vi "LabviewV4.vi"() -> ()   [LabVIEW 2010]
uses:
  <vilib>/Instr/_visa.llb/VISA Configure Serial Port (Instr).vi
panel:
  in  "Registar tensão":bool
  in  "Posição de destino da bola (Set Point)":i16
  out "Instruções":string="HOME X Y\r\n" caption="Instruções para traçar gráfico"
  out "Mensagem enviada":string="HOME X Y\r\n"
  out "read string":string caption="Recebido"
  in  "delay before read (ms)":u32=500
  in  "stop":bool
  in  "VISA Resource Name":refnum<visa-resource-name>
  # "Bola na calha"
  # "Posição limite esquerda = -150 Posição limite direita = 150\nValores inseridos fora do intervalo acima contam como o limite mais próximo do digitado"
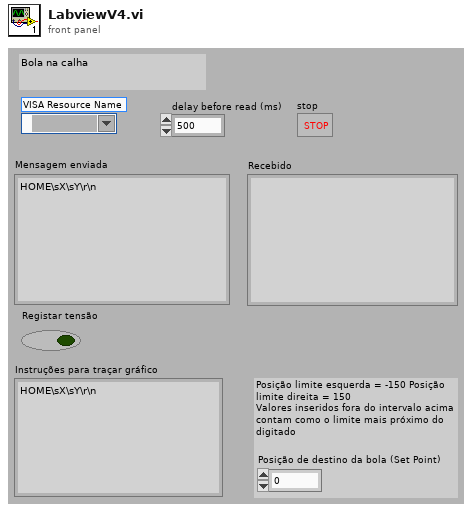
[diagram p1: front panel]
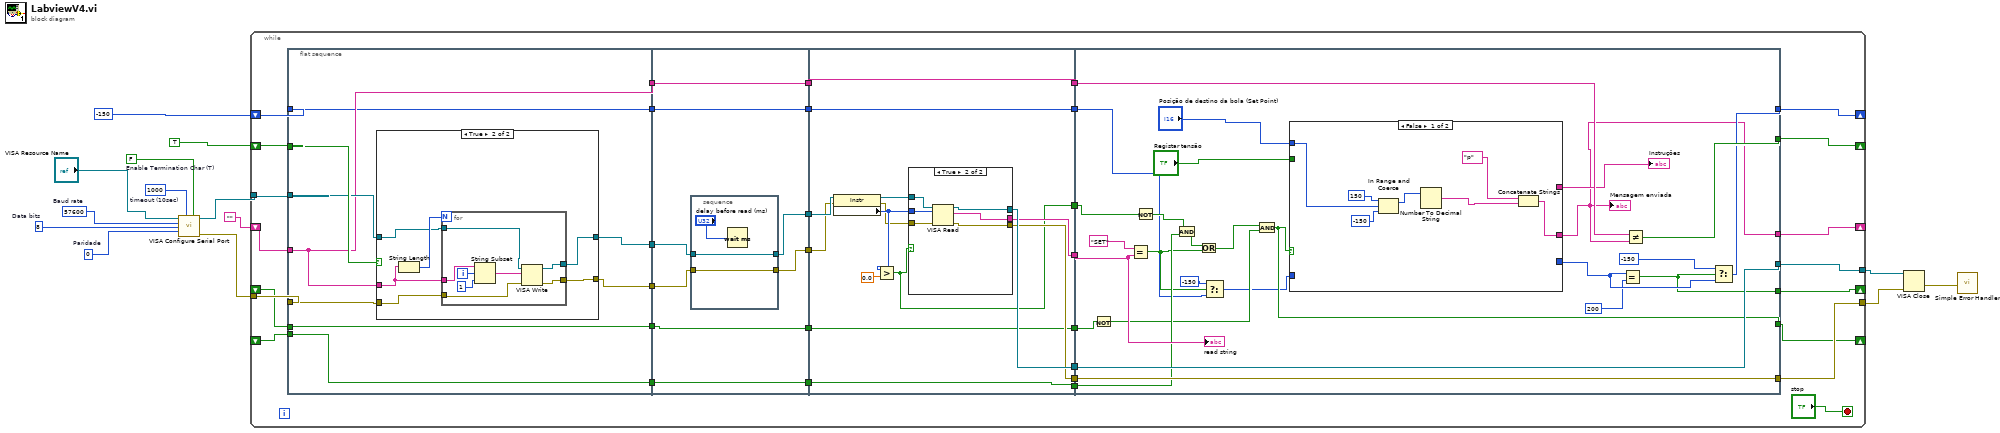
[diagram p0: block diagram]
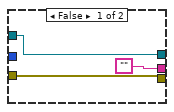
[diagram p3: hidden frame]
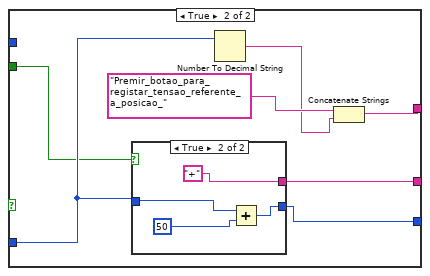
[diagram p4: hidden frame]
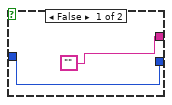
[diagram p5: hidden frame]
diagram:
  w10 = u32 0  # Paridade
  w11 = u32 8  # Data bits
  w12 = u32 57600  # Baud rate
  w13 = FALSE  # Enable Termination Char (T)
  w14 = u32 1000  # timeout (10sec)
  n1 = call-poly "VISA Configure Serial Port"("VISA resource name"="VISA Resource Name", "timeout (10sec)"=w14, "Enable Termination\nChar (T)"=w13, "baud rate (9600)"=w12, "data bits (8)"=w11, "parity (0:none)"=w10) -> ("VISA resource name out"=w5:refnum<visa-resource-name>, "error out"=w6:errorcluster)  [unwired: 8 in]
  n2 = while {
    shift-right: [w42] -> _
    shift-left: "" -> [w46]
    shift-right: [w34] -> _
    shift-left: i16 -150 ("Numeric 2") -> [w35]
    tunnel: w6 -> [w47]
    tunnel: w5 -> [w48]
    shift-right: [w41] -> _
    shift-left: TRUE -> [w39]
    tunnel: [w31] -> w2
    tunnel: [w30] -> w1
    shift-right: [w25] -> _
    shift-left: _ -> [w24]
    shift-right: [w19] -> _
    shift-left: _ -> [w17]
    stop <- "stop" stop-if-true
    n3 = flat-sequence {
      tunnel: w48 -> [w57]
      tunnel: w47 -> [w56]
      tunnel: w46 -> [w53]
      tunnel: [w55] -> w45
      tunnel: w39 -> [w58]
      tunnel: [w50] -> w36
      tunnel: w35 -> [w50]
      tunnel: [w54] -> w29
      tunnel: [w53] -> w26
      tunnel: w24 -> [w52]
      tunnel: [w52] -> w21
      tunnel: [w51] -> w18
      tunnel: w17 -> [w51]
      tunnel: w45 -> [w82]
      tunnel: [w80] -> w44
      tunnel: [w79] -> w43
      tunnel: [w78] -> w37
      tunnel: w36 -> [w78]
      tunnel: w29 -> [w81]
      tunnel: [w77] -> w27
      tunnel: w26 -> [w77]
      tunnel: [w76] -> w22
      tunnel: w21 -> [w76]
      tunnel: w18 -> [w75]
      tunnel: [w75] -> w15
      tunnel: w44 -> [w93]
      tunnel: w43 -> [w94]
      tunnel: [w90] -> w40
      tunnel: [w99] -> w38
      tunnel: w37 -> [w99]
      tunnel: [w91] -> w33
      tunnel: [w92] -> w32
      tunnel: [w89] -> w28
      tunnel: w27 -> [w89]
      tunnel: [w88] -> w23
      tunnel: w22 -> [w88]
      tunnel: [w87] -> w20
      tunnel: [w86] -> w16
      tunnel: w15 -> [w86]
      tunnel: [w109] -> w42
      tunnel: [w132] -> w41
      tunnel: w40 -> [w124]
      tunnel: w38 -> [w111]
      tunnel: [w130] -> w34
      tunnel: w33 -> [w129]
      tunnel: w32 -> [w128]
      tunnel: [w129] -> w31
      tunnel: [w128] -> w30
      tunnel: w28 -> [w127]
      tunnel: [w115] -> w25
      tunnel: w23 -> [w123]
      tunnel: w20 -> [w121]
      tunnel: [w119] -> w19
      tunnel: w16 -> [w117]
      frame #0 {
        n4 = case shown="True" w58 {
          tunnel: [w59 w66] -> w54
          tunnel: [w60 w65] -> w55
          tunnel: w53 -> [_ w63]
          tunnel: w57 -> [w60 w62]
          tunnel: w56 -> [w59 w61]
          frame False {
          }
          frame True {
            n5 = String Length(string=w63) -> (length=w64:i32)
            n6 = for {
              N: w64 -> [_]
              tunnel: [w74] -> w66
              tunnel: [w73] -> w65
              tunnel: w63 -> [w72]
              tunnel: w62 -> [w69]
              tunnel: w61 -> [w68]
              i -> [w67]
              n7 = String Subset(string=w72, offset (0)=w67, length (rest)=1 ("length (rest)")) -> (substring=w71:string)
              n8 = VISA Write(VISA resource name=w69, write buffer=w71, error in (no error)=w68) -> (VISA resource name out=w73:refnum<visa-resource-name>, error out=w74:errorcluster)  [unwired: 1 out]
            }
          }
        }
      }
      frame #1 {
        n9 = stacked-sequence {
          tunnel: w81 -> [w85]
          tunnel: [w85] -> w80
          tunnel: w82 -> [w84]
          tunnel: [w84] -> w79
          frame #0 {
            n10 = Wait (ms)(milliseconds to wait="delay before read (ms)") -> ()  [unwired: 1 out]
          }
        }
      }
      frame #2 {
        n11 = property class="Instr"(reference=w94, error in=w93) -> (reference out=w96:refnum<visa-resource-name>, error out=w95:errorcluster, "Serial Settings:Number of Bytes at Serial Port"=w98:u32)
        n12 = Greater?(x=w98, y=0.0 ("x")) -> (0:w87:bool)
        n13 = case shown="True" w87 {
          tunnel: [w102 w106] -> w91
          tunnel: [w101 w108] -> w92
          tunnel: ["" w107] -> w90
          tunnel: w98 -> [_ w105]
          tunnel: w95 -> [w102 w104]
          tunnel: w96 -> [w101 w103]
          frame False {
          }
          frame True {
            n14 = VISA Read(VISA resource name=w103, byte count=w105, error in (no error)=w104) -> (VISA resource name out=w108:refnum<visa-resource-name>, read buffer=w107:string, error out=w106:errorcluster)  [unwired: 1 out]
          }
        }
      }
      frame #3 {
        n15 = Not(x=w117) -> (.not. x?=w116:bool)
        n16 = Equal?(x="SET" ("Resultado 2"), y=w124) -> (x = y?=w112:bool)
        n17 = Not(x=w121) -> (.not. x?=w120:bool)
        n18 = And(x=w120, y=w123) -> (x .and. y?=w122:bool)
        n19 = Or(x=w122, y=w112) -> (x .or. y?=w118:bool)
        n20 = Select(t=-150 ("Numeric 2"), s=w112, f=w111) -> (s? t:f=w110:i32)
        n21 = And(x=w118, y=w116) -> (x .and. y?=w115:bool)
        n22 = case shown="False" w115 {
          tunnel: "Posição de destino da bola (Set Point)" -> [w141 _]
          tunnel: w110 -> [_ w149]
          tunnel: [u8 0 ("Numeric 2") w144] -> w135
          tunnel: [w136 w147] -> w109
          tunnel: [_ w146] -> w126
          tunnel: "Registar tensão" -> [_ w145]
          frame False {
            n23 = In Range and Coerce(upper limit=i16 150, x=w141, lower limit=i16 -150) -> (coerced(x)=w139:i16)  [unwired: 1 out]
            n24 = Number To Decimal String(number=w139) -> (decimal integer string=w138:string)  [unwired: 1 in]
            n25 = Concatenate Strings("p" ("Resultado 2"), w138) -> (w136:string)
          }
          frame True {
            n26 = case shown="True" w145 {
              tunnel: w149 -> [w152 w155]
              tunnel: [w152 w154] -> w144
              tunnel: ["" "+" ("Resultado 2")] -> w147
              frame False {
              }
              frame True {
                n27 = Add(x=w155, y=50 ("Numeric 2")) -> (x+y=w154:i32)
              }
            }
            n28 = Number To Decimal String(number=w149) -> (decimal integer string=w148:string)  [unwired: 1 in]
            n29 = Concatenate Strings("Premir_botao_para_registar_tensao_referente_a_posicao_" ("Resultado 2"), w148) -> (w146:string)
          }
        }
        "Instruções" <- w126
        "Mensagem enviada" <- w109
        n30 = Equal?(x=w135, y=i16 200 ("Numeric 2")) -> (x = y?=w119:bool)
        n31 = Not Equal?(x=w127, y=w109) -> (x != y?=w132:bool)
        n32 = Select(t=-150 ("Numeric 2"), s=w119, f=w135) -> (s? t:f=w130:i32)
        "read string" <- w124
      }
    }
  }
  n33 = VISA Close(VISA resource name=w1, error in (no error)=w2) -> (error out=w8:errorcluster)
  n34 = call <vilib>:"Simple Error Handler.vi"("error in (no error)"=w8) -> ()  [unwired: 4 in, 5 out]
